vi "SimpleLiveAppColor.vi"() -> ()   [LabVIEW 2018]
uses:
  D:/SVN/PM/sdk/AppSamples/LabVIEWSamples/trunk/Release/2018/Dependencies/PVCamNET.dll
  Dependencies/PVCamNET.dll
panel:
  in  "Color":bool
  out "Name":string
  in  "Bayer pattern":string(combo)
  in  "Exposure Time":dbl
  in  "Live":bool
  in  "Camera Status":bool
  in  "Uninit":bool
  in  "Live stop":bool
  in  "Live start":bool
  in  "Init":bool
  # "SimpleLiveAppColor.vi\n\nDescription:\nThis sample code lets the user use color mode for a supported camera\n in an event driven structure.\n\nSteps to run:\n1. Click \"Run\"\n2. Click \"Open\"\n3. Enter Exposure Time\n4. Toggle Color switch\n5. Click \"Live start\"\n6. Click \"Live stop\"\n7. Click \"Close\""
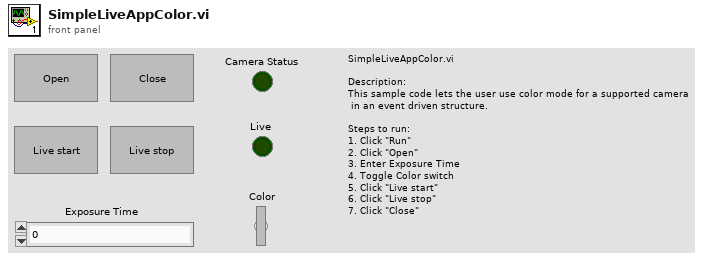
[diagram p1: front panel]
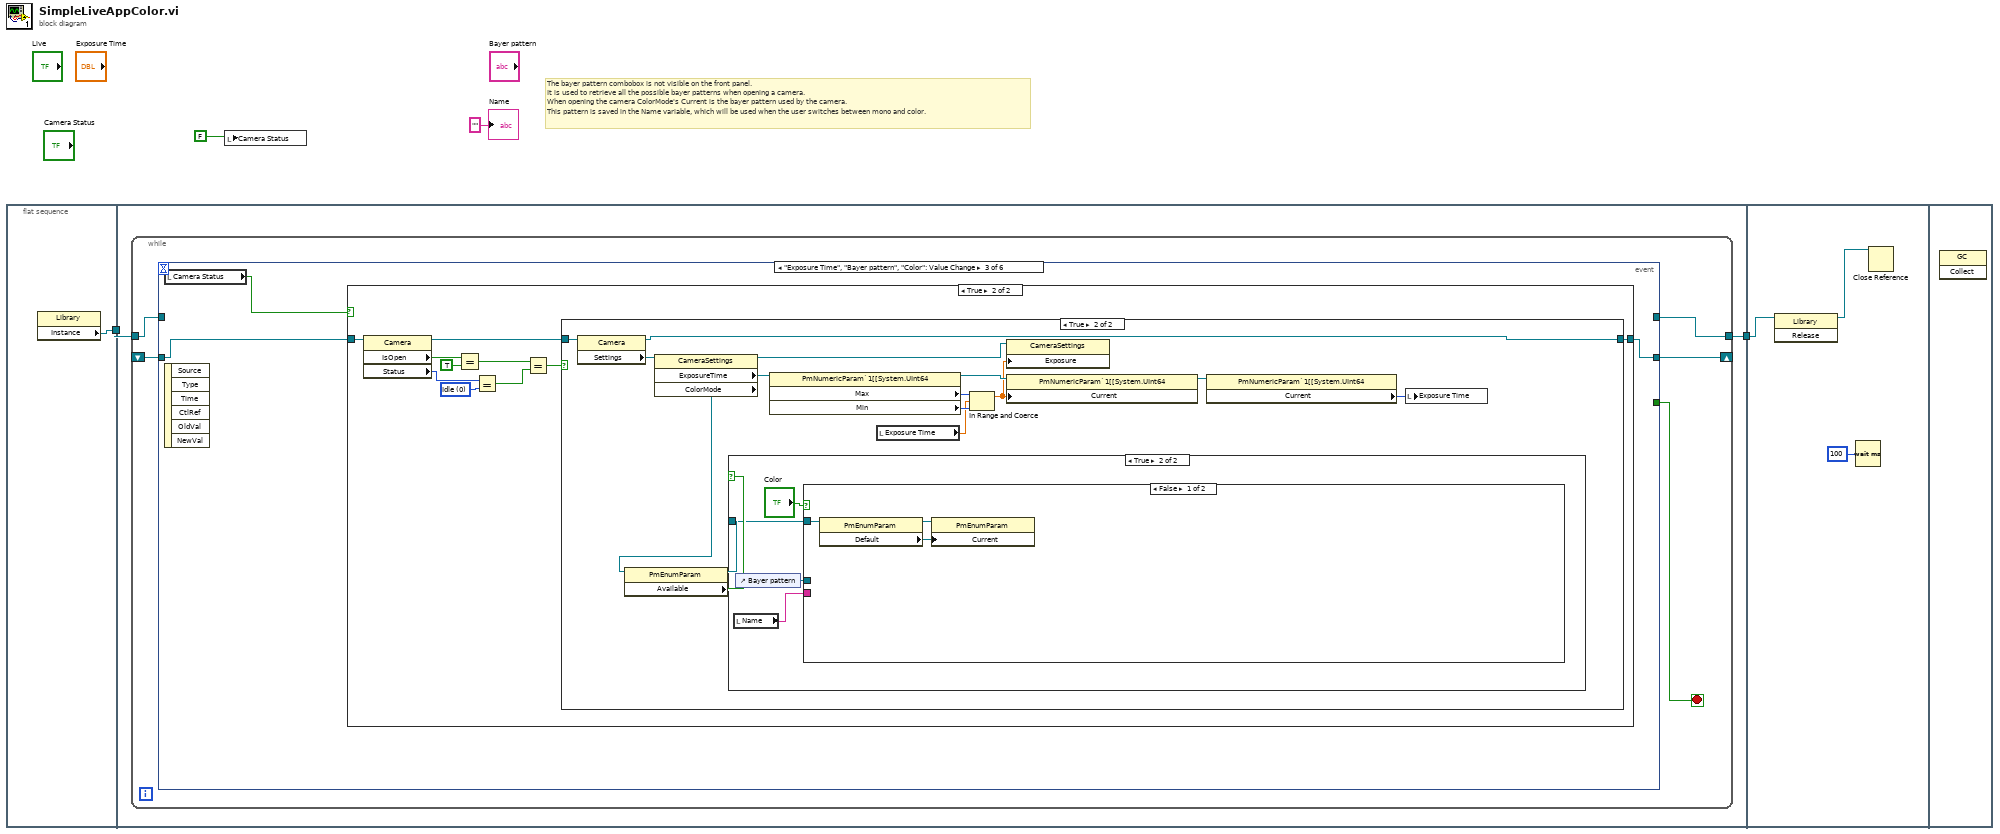
[diagram p0: block diagram]
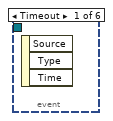
[diagram p2: hidden frame]
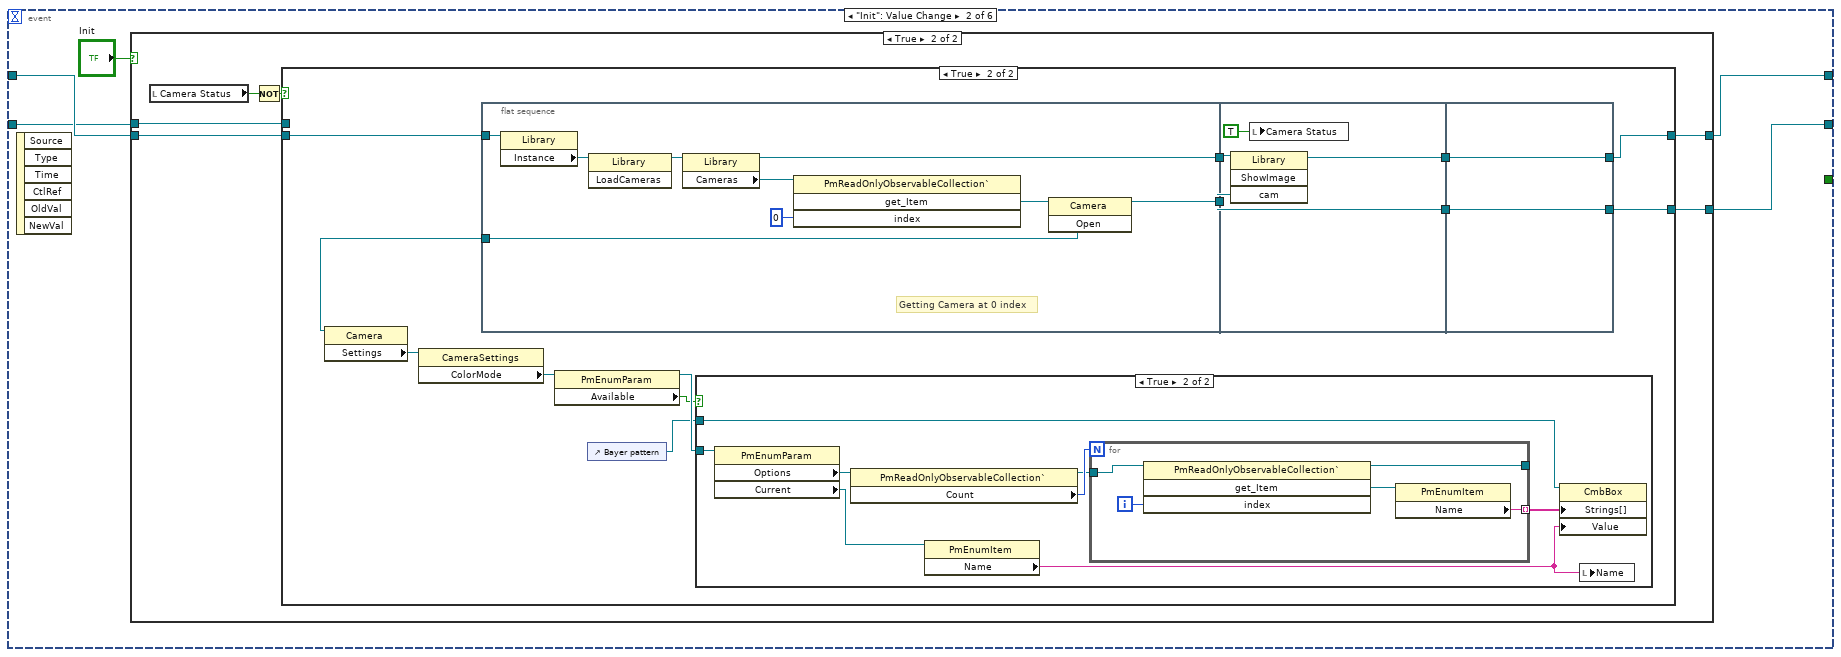
[diagram p3: hidden frame]
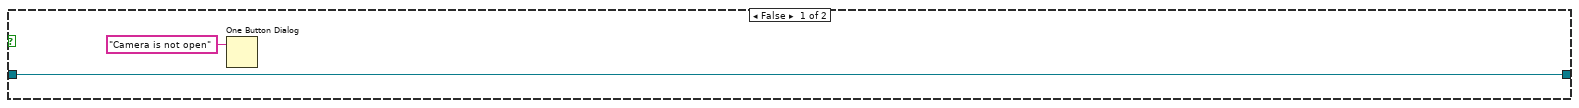
[diagram p7: hidden frame]
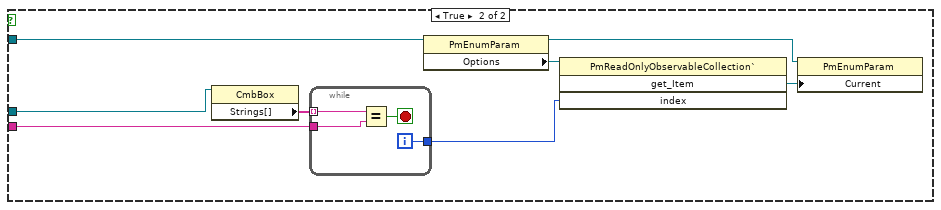
[diagram p10: hidden frame]
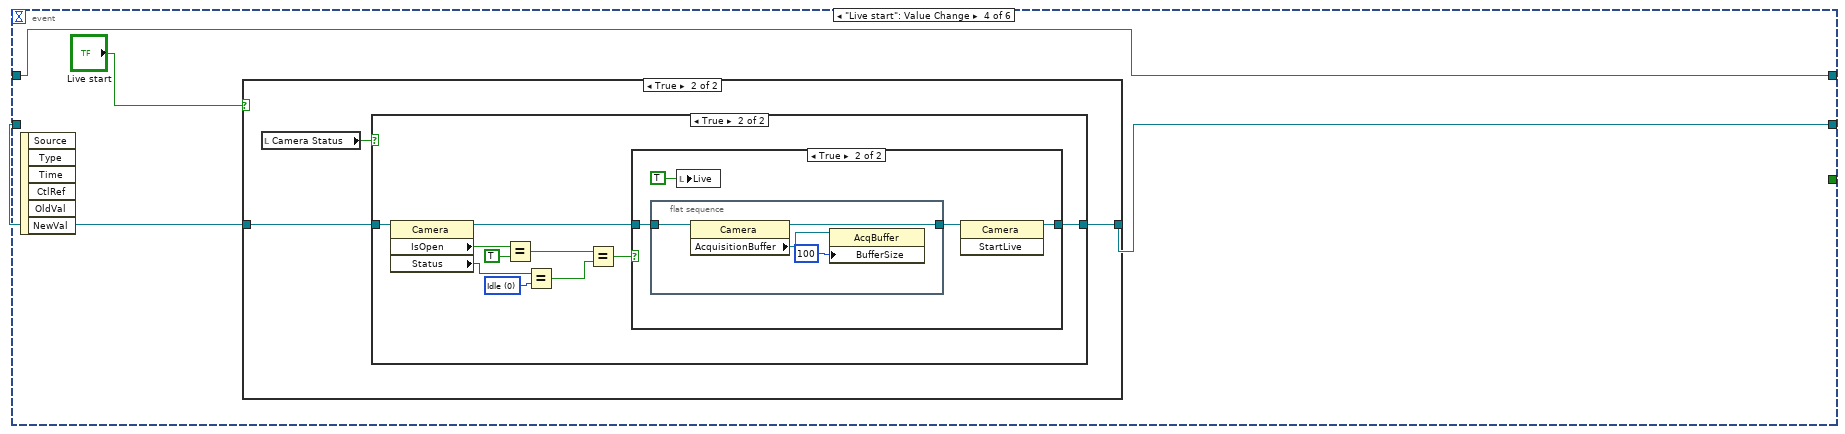
[diagram p11: hidden frame]
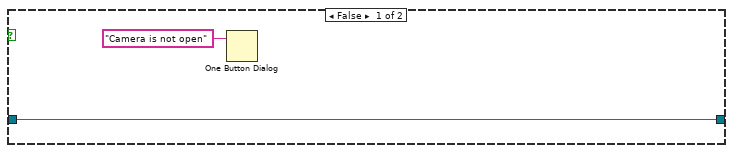
[diagram p13: hidden frame]
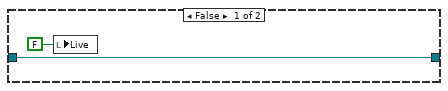
[diagram p14: hidden frame]
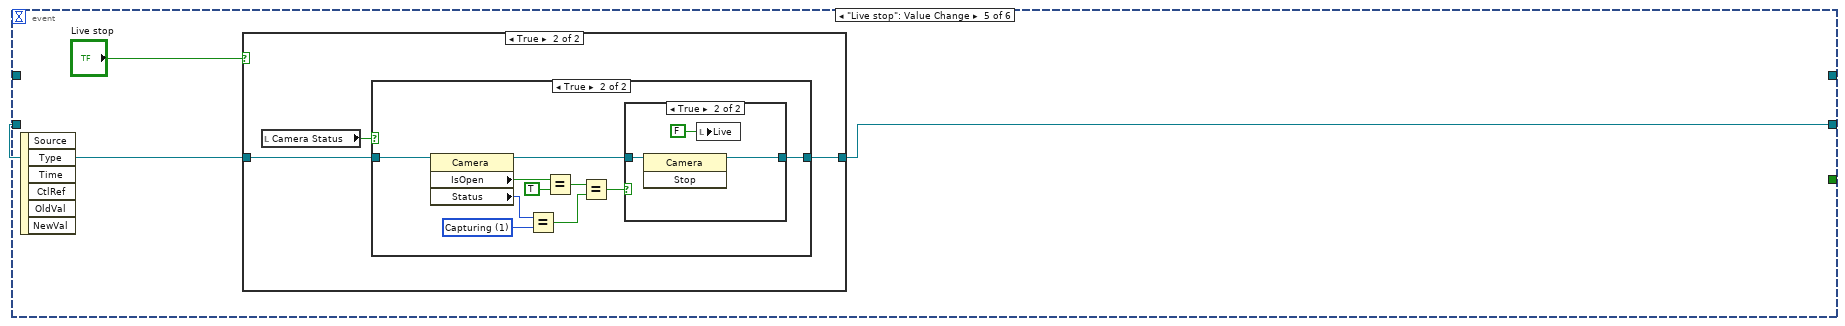
[diagram p15: hidden frame]
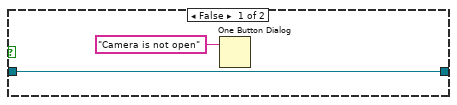
[diagram p17: hidden frame]
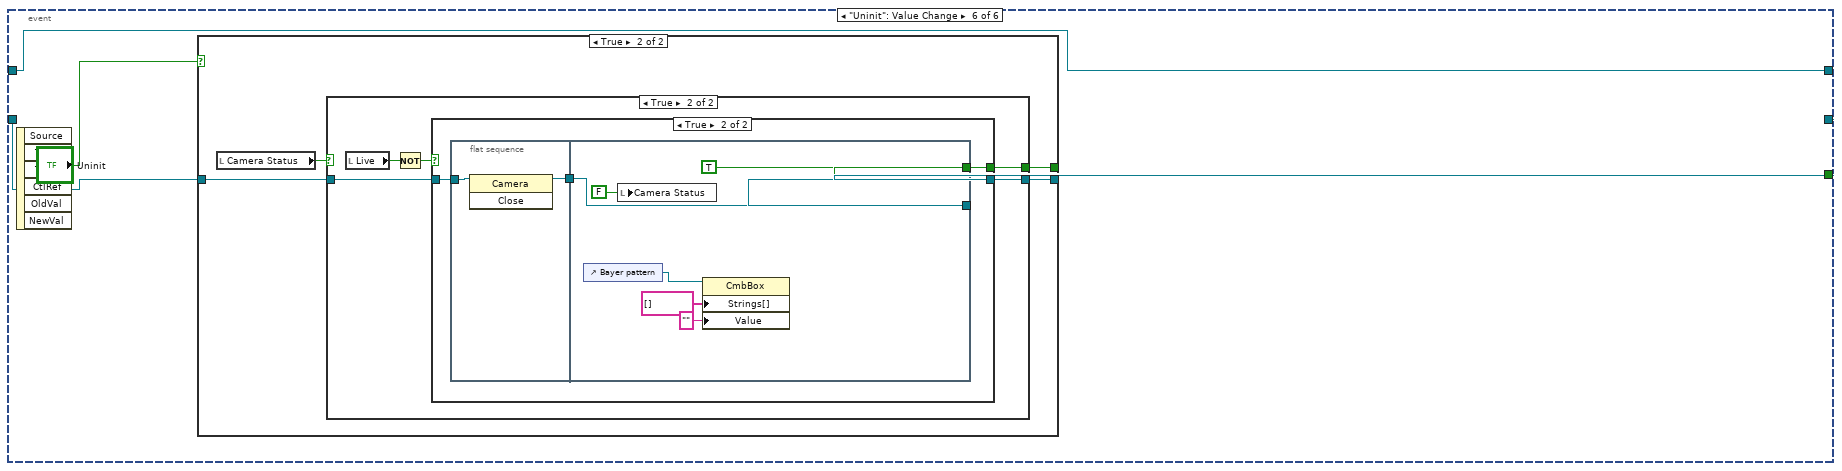
[diagram p19: hidden frame]
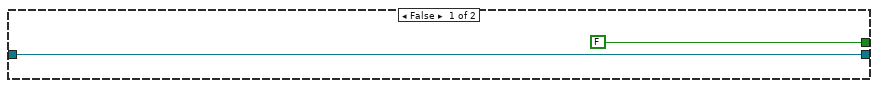
[diagram p20: hidden frame]
diagram:
  # "The bayer pattern combobox is not visible on the front panel.\nIt is used to retrieve all the possible bayer patterns when opening a camera.\nWhen opening the camera ColorMode's Current is the bayer pattern used by the camera.\nThis pattern is saved in the Name variable, which will be used when the user switches between mono and color."
  n1 = flat-sequence {
    tunnel: [w5] -> w4
    tunnel: w4 -> [w7]
    tunnel: [w6] -> w3
    tunnel: w3 -> [w205]
    frame #0 {
      n2 = property class="Library"() -> ("Instance"=w5:refnum<k24>)  [unwired: 2 in, 2 out]
    }
    frame #1 {
      n3 = while {
        tunnel: w7 -> [w12]
        shift-right: [w11] -> _
        shift-left: _ -> [w9]
        tunnel: [w10] -> w6
        stop <- w8 stop-if-true
        n4 = event shown="[2] \"Exposure Time\", \"Bayer pattern\", \"Color\": Value Change" {
          selector: _ -> [_ _ _ _ _ _]
          dyn-events: _ -> [_ _ _ _ _ _]
          timeout: _ -> [_ _ _ _ _ _]
          tunnel: w12 -> [_ w17 w69 w119 _ w174]
          tunnel: [_ w16 w70 w120 w149 w175] -> w11
          tunnel: [_ w15 w69 w119 _ w174] -> w10
          tunnel: w9 -> [_ w14 w71 w121 w150 w176]
          tunnel: [_ _ _ _ _ w173] -> w8
          event Timeout {
            n5 = event-data() -> ()  [unwired: 1 in, 3 out]
          }
          event "Init": Value Change {
            n6 = event-data() -> ()  [unwired: 1 in, 6 out]
            n7 = case shown="True" "Init" {
              tunnel: w17 -> [w19 w25]
              tunnel: [w18 w24] -> w16
              tunnel: [w19 w23] -> w15
              tunnel: w14 -> [w18 w20]
              frame False {
              }
              frame True {
                n8 = local read "Camera Status"() -> (w22:bool)
                n9 = Not(x=w22) -> (.not. x?=w21:bool)
                n10 = case shown="True" w21 {
                  tunnel: w25 -> [w26 w38]
                  tunnel: [w27 w37] -> w24
                  tunnel: [w26 w36] -> w23
                  tunnel: w20 -> [w27 _]
                  frame False {
                  }
                  frame True {
                    n11 = property class="Camera"(reference=w28) -> ("Settings"=w29:refnum<k24>)  [unwired: 1 in, 2 out]
                    n12 = property class="CameraSettings"(reference=w29) -> ("ColorMode"=w30:refnum<k24>)  [unwired: 1 in, 2 out]
                    n13 = flat-sequence {
                      tunnel: w38 -> [w57]
                      tunnel: [w58] -> w40
                      tunnel: [w54] -> w39
                      tunnel: [w54] -> w28
                      tunnel: w40 -> [w64]
                      tunnel: w39 -> [w65]
                      tunnel: [w65] -> w35
                      tunnel: [w63] -> w34
                      tunnel: [w66] -> w36
                      tunnel: [w67] -> w37
                      tunnel: w35 -> [w67]
                      tunnel: w34 -> [w66]
                      frame #0 {
                        # "Getting Camera at 0 index"
                        n14 = property class="Library"(reference=w57) -> ("Instance"=w56:refnum<k24>)  [unwired: 1 in, 2 out]
                        n15 = invoke class="Library" method="LoadCameras"(reference=w56) -> (reference out=w55:refnum<k24>)  [unwired: 2 in, 2 out]
                        n16 = property class="Library"(reference=w55) -> (reference out=w58:refnum<k24>, "Cameras"=w61:refnum<k24>)  [unwired: 1 in, 1 out]
                        n17 = invoke class="PmReadOnlyObservableCollection`" method="get_Item"(reference=w61, "index"=0) -> ("get_Item"=w59:refnum<k24>)  [unwired: 2 in, 3 out]
                        n18 = invoke class="Camera" method="Open"(reference=w59) -> (reference out=w54:refnum<k24>)  [unwired: 2 in, 2 out]
                      }
                      frame #1 {
                        n19 = invoke class="Library" method="ShowImage"(reference=w64, "cam"=w65) -> (reference out=w63:refnum<k24>)  [unwired: 2 in, 3 out]
                        n20 = local write "Camera Status"(TRUE ("Camera Status")) -> ()
                      }
                      frame #2 {
                      }
                    }
                    n21 = property class="PmEnumParam"(reference=w30) -> (reference out=w33:refnum<k24>, "Available"=w32:bool)  [unwired: 1 in, 1 out]
                    n22 = control-ref of="Bayer pattern"() -> (w31:refnum<vi>)
                    n23 = case shown="True" w32 {
                      tunnel: w31 -> [_ w47]
                      tunnel: w33 -> [_ w46]
                      frame False {
                      }
                      frame True {
                        n24 = property class="PmEnumParam"(reference=w46) -> ("Options"=w45:refnum<k24>, "Current"=w42:refnum<k24>)  [unwired: 1 in, 2 out]
                        n25 = property class="PmReadOnlyObservableCollection`"(reference=w45) -> (reference out=w43:refnum<k24>, "Count"=w44:i32)  [unwired: 1 in, 1 out]
                        n26 = property class="PmEnumItem"(reference=w42) -> ("Name"=w41:string)  [unwired: 1 in, 2 out]
                        n27 = for {
                          N: w44 -> [_]
                          tunnel: [w53] -> w48 mode=indexing
                          tunnel: [w49] -> _
                          tunnel: w43 -> [w52]
                          i -> [w51]
                          n28 = invoke class="PmReadOnlyObservableCollection`" method="get_Item"(reference=w52, "index"=w51) -> (reference out=w49:refnum<k24>, "get_Item"=w50:refnum<k24>)  [unwired: 2 in, 2 out]
                          n29 = property class="PmEnumItem"(reference=w50) -> ("Name"=w53:string)  [unwired: 1 in, 2 out]
                        }
                        n30 = property class="CmbBox"(reference=w47, "Strings[]"=w48, "Value"=w41) -> ()  [unwired: 1 in, 2 out]
                        n31 = local write "Name"(w41) -> ()
                      }
                    }
                  }
                }
              }
            }
          }
          event "Exposure Time", "Bayer pattern", "Color": Value Change {
            n32 = local read "Camera Status"() -> (w68:bool)
            n33 = event-data() -> ()  [unwired: 1 in, 6 out]
            n34 = case shown="True" w68 {
              tunnel: w71 -> [w73 w77]
              tunnel: [w73 w74] -> w70
              frame False {
                n35 = One Button Dialog(message="Camera is not open") -> ()  [unwired: 1 in, 1 out]
              }
              frame True {
                w82 = 0 items=["Idle", "Capturing"] ("Status")
                n36 = property class="Camera"(reference=w77) -> (reference out=w75:refnum<k24>, "IsOpen"=w81:bool, "Status"=w83:i32)  [unwired: 1 in, 1 out]
                n37 = Equal?(x=w81, y=TRUE) -> (x = y?=w79:bool)
                n38 = Equal?(x=w83, y=w82) -> (x = y?=w78:bool)
                n39 = Equal?(x=w79, y=w78) -> (x = y?=w76:bool)
                n40 = case shown="True" w76 {
                  tunnel: w75 -> [w84 w99]
                  tunnel: [w84 w88] -> w74
                  frame False {
                  }
                  frame True {
                    n41 = property class="Camera"(reference=w99) -> (reference out=w88:refnum<k24>, "Settings"=w98:refnum<k24>)  [unwired: 1 in, 1 out]
                    n42 = property class="CameraSettings"(reference=w98) -> (reference out=w91:refnum<k24>, "ExposureTime"=w92:refnum<k24>, "ColorMode"=w86:refnum<k24>)  [unwired: 1 in, 1 out]
                    n43 = property class="PmEnumParam"(reference=w86) -> (reference out=w85:refnum<k24>, "Available"=w87:bool)  [unwired: 1 in, 1 out]
                    n44 = case shown="True" w87 {
                      tunnel: w85 -> [_ w103]
                      frame False {
                      }
                      frame True {
                        n45 = local read "Name"() -> (w100:string)
                        n46 = control-ref of="Bayer pattern"() -> (w101:refnum<vi>)
                        n47 = case shown="False" "Color" {
                          tunnel: w103 -> [w106 w113]
                          tunnel: w101 -> [_ w108]
                          tunnel: w100 -> [_ w107]
                          frame False {
                            n48 = property class="PmEnumParam"(reference=w106) -> (reference out=w104:refnum<k24>, "Default"=w105:refnum<k24>)  [unwired: 1 in, 1 out]
                            n49 = property class="PmEnumParam"(reference=w104, "Current"=w105) -> ()  [unwired: 1 in, 2 out]
                          }
                          frame True {
                            n50 = property class="CmbBox"(reference=w108) -> ("Strings[]"=w114:string[])  [unwired: 1 in, 2 out]
                            n51 = while {
                              tunnel: w114 -> [w118] mode=indexing
                              tunnel: [w116] -> w111
                              tunnel: w107 -> [w115]
                              i -> [w116]
                              stop <- w117 stop-if-true
                              n52 = Equal?(x=w118, y=w115) -> (x = y?=w117:bool)
                            }
                            n53 = property class="PmEnumParam"(reference=w113) -> (reference out=w109:refnum<k24>, "Options"=w112:refnum<k24>)  [unwired: 1 in, 1 out]
                            n54 = invoke class="PmReadOnlyObservableCollection`" method="get_Item"(reference=w112, "index"=w111) -> ("get_Item"=w110:refnum<k24>)  [unwired: 2 in, 3 out]
                            n55 = property class="PmEnumParam"(reference=w109, "Current"=w110) -> ()  [unwired: 1 in, 2 out]
                          }
                        }
                      }
                    }
                    n56 = property class="PmNumericParam`1[[System.UInt64"(reference=w92) -> (reference out=w95:refnum<k24>, "Max"=w97:u64, "Min"=w96:u64)  [unwired: 1 in, 1 out]
                    n57 = local read "Exposure Time"() -> (w90:dbl)
                    n58 = In Range and Coerce(upper limit=w97, x=w90, lower limit=w96) -> (coerced(x)=w93:dbl)  [unwired: 1 out]
                    n59 = property class="CameraSettings"(reference=w91, "Exposure"=w93) -> ()  [unwired: 1 in, 2 out]
                    n60 = property class="PmNumericParam`1[[System.UInt64"(reference=w95, "Current"=w93) -> (reference out=w94:refnum<k24>)  [unwired: 1 in, 1 out]
                    n61 = property class="PmNumericParam`1[[System.UInt64"(reference=w94) -> ("Current"=w89:u64)  [unwired: 1 in, 2 out]
                    n62 = local write "Exposure Time"(w89) -> ()
                  }
                }
              }
            }
          }
          event "Live start": Value Change {
            n63 = event-data() -> ()  [unwired: 1 in, 6 out]
            n64 = case shown="True" "Live start" {
              tunnel: w121 -> [w123 w126]
              tunnel: [w123 w125] -> w120
              frame False {
              }
              frame True {
                n65 = local read "Camera Status"() -> (w124:bool)
                n66 = case shown="True" w124 {
                  tunnel: w126 -> [w127 w132]
                  tunnel: [w127 w130] -> w125
                  frame False {
                    n67 = One Button Dialog(message="Camera is not open") -> ()  [unwired: 1 in, 1 out]
                  }
                  frame True {
                    w137 = 0 items=["Idle", "Capturing"] ("Status")
                    n68 = property class="Camera"(reference=w132) -> (reference out=w131:refnum<k24>, "IsOpen"=w136:bool, "Status"=w138:i32)  [unwired: 1 in, 1 out]
                    n69 = Equal?(x=w136, y=TRUE) -> (x = y?=w134:bool)
                    n70 = Equal?(x=w138, y=w137) -> (x = y?=w133:bool)
                    n71 = Equal?(x=w134, y=w133) -> (x = y?=w129:bool)
                    n72 = case shown="True" w129 {
                      tunnel: w131 -> [w140 w142]
                      tunnel: [w140 w143] -> w130
                      frame False {
                        n73 = local write "Live"(FALSE ("Live 2")) -> ()
                      }
                      frame True {
                        n74 = flat-sequence {
                          tunnel: w142 -> [w148]
                          tunnel: [w145] -> w141
                          frame #0 {
                            n75 = property class="Camera"(reference=w148) -> (reference out=w145:refnum<k24>, "AcquisitionBuffer"=w147:refnum<k24>)  [unwired: 1 in, 1 out]
                            n76 = property class="AcqBuffer"(reference=w147, "BufferSize"=100) -> ()  [unwired: 1 in, 2 out]
                          }
                        }
                        n77 = local write "Live"(TRUE ("Live")) -> ()
                        n78 = invoke class="Camera" method="StartLive"(reference=w141) -> (reference out=w143:refnum<k24>)  [unwired: 2 in, 2 out]
                      }
                    }
                  }
                }
              }
            }
          }
          event "Live stop": Value Change {
            n79 = event-data() -> ()  [unwired: 1 in, 6 out]
            n80 = case shown="True" "Live stop" {
              tunnel: w150 -> [w152 w155]
              tunnel: [w152 w154] -> w149
              frame False {
              }
              frame True {
                n81 = local read "Camera Status"() -> (w153:bool)
                n82 = case shown="True" w153 {
                  tunnel: w155 -> [w157 w167]
                  tunnel: [w157 w164] -> w154
                  frame False {
                    n83 = One Button Dialog(message="Camera is not open") -> ()  [unwired: 1 in, 1 out]
                  }
                  frame True {
                    w162 = 1 items=["Idle", "Capturing"] ("Status")
                    n84 = property class="Camera"(reference=w167) -> (reference out=w165:refnum<k24>, "IsOpen"=w161:bool, "Status"=w163:i32)  [unwired: 1 in, 1 out]
                    n85 = Equal?(x=w163, y=w162) -> (x = y?=w158:bool)
                    n86 = Equal?(x=w161, y=TRUE) -> (x = y?=w159:bool)
                    n87 = Equal?(x=w159, y=w158) -> (x = y?=w166:bool)
                    n88 = case shown="True" w166 {
                      tunnel: w165 -> [w168 w171]
                      tunnel: [w168 w170] -> w164
                      frame False {
                      }
                      frame True {
                        n89 = invoke class="Camera" method="Stop"(reference=w171) -> (reference out=w170:refnum<k24>)  [unwired: 2 in, 2 out]
                        n90 = local write "Live"(FALSE ("Live 2")) -> ()
                      }
                    }
                  }
                }
              }
            }
          }
          event "Uninit": Value Change {
            n91 = event-data() -> ()  [unwired: 1 in, 6 out]
            n92 = case shown="True" "Uninit" {
              tunnel: w176 -> [w178 w182]
              tunnel: [w178 w181] -> w175
              tunnel: [FALSE ("Camera Status") w179] -> w173
              frame False {
              }
              frame True {
                n93 = local read "Camera Status"() -> (w180:bool)
                n94 = case shown="True" w180 {
                  tunnel: w182 -> [w184 w189]
                  tunnel: [w184 w188] -> w181
                  tunnel: [FALSE ("Camera Status") w187] -> w179
                  frame False {
                  }
                  frame True {
                    n95 = local read "Live"() -> (w185:bool)
                    n96 = Not(x=w185) -> (.not. x?=w186:bool)
                    n97 = case shown="True" w186 {
                      tunnel: w189 -> [w191 w194]
                      tunnel: [w191 w193] -> w188
                      tunnel: [FALSE ("Camera Status") w192] -> w187
                      frame False {
                      }
                      frame True {
                        n98 = flat-sequence {
                          tunnel: w194 -> [w197]
                          tunnel: [w196] -> w195
                          tunnel: [w203] -> w193
                          tunnel: w195 -> [w203]
                          tunnel: [TRUE ("Camera Status")] -> w192
                          frame #0 {
                            n99 = invoke class="Camera" method="Close"(reference=w197) -> (reference out=w196:refnum<k24>)  [unwired: 2 in, 2 out]
                          }
                          frame #1 {
                            n100 = control-ref of="Bayer pattern"() -> (w200:refnum<vi>)
                            n101 = local write "Camera Status"(FALSE ("Camera Status")) -> ()
                            n102 = property class="CmbBox"(reference=w200, "Strings[]"=string[] [] ("Strings []"), "Value"="") -> ()  [unwired: 1 in, 2 out]
                          }
                        }
                      }
                    }
                  }
                }
              }
            }
          }
        }
      }
    }
    frame #2 {
      n103 = invoke class="Library" method="Release"(reference=w205) -> (reference out=w206:refnum<k24>)  [unwired: 2 in, 2 out]
      n104 = Wait (ms)(milliseconds to wait=u32 100) -> ()  [unwired: 1 out]
      n105 = Close Reference(reference=w206) -> ()  [unwired: 1 in, 1 out]
    }
    frame #3 {
      n106 = invoke class="GC" method="Collect"() -> ()  [unwired: 3 in, 3 out]
    }
  }
  n107 = local write "Camera Status"(FALSE ("Camera Status")) -> ()
  "Name" <- "" ("Name")
